vi "PROGRAMA.vi"() -> ()   [LabVIEW 2011]
doc: "Read one the value of one analog channel from a LINX device."
uses:
  <vilib>/Platform/TimedLoop/XDataNode/timing_clust.ctl
  <vilib>/Platform/TimedLoop/XDataNode/nitl_modes.ctl
  <vilib>/Platform/TimedLoop/XDataNode/wakeup.ctl
  <vilib>/MakerHub/LINX/Public/Peripherals/Analog/Analog Read 1 Chan.vi
  <vilib>/MakerHub/LINX/Public/Peripherals/PWM/PWM Set Duty Cycle 1 Chan.vi
  <vilib>/MakerHub/LINX/Public/Peripherals/Digital/Digital Write 1 Chan.vi
  <vilib>/MakerHub/LINX/Public/Peripherals/Analog/Analog Read N Chans.vi
  <vilib>/MakerHub/LINX/Public/Peripherals/Digital/Digital Write N Chans.vi
  <vilib>/MakerHub/LINX/Private/Local IO/LinxAnalogRead.vi
  <vilib>/MakerHub/LINX/Public/Utilities/Check Channel.vi
  <vilib>/MakerHub/LINX/Private/Local IO/LinxDigitalWrite.vi
  <vilib>/MakerHub/LINX/Public/Utilities/Open Serial.vi
  <vilib>/addons/Fuzzy Logic/FL Fuzzy Controller (SISO).vi
  <vilib>/addons/Fuzzy Logic/FL Fuzzy Controller (SIMO).vi
  <vilib>/addons/control/pid/pid.llb/PID (DBL).vi
  <vilib>/Utility/file.llb/Write To Spreadsheet File (string).vi
  <vilib>/MakerHub/LINX/Private/Utilties/Generate Error.vi
  <vilib>/Utility/file.llb/Read From Spreadsheet File (DBL).vi
  <vilib>/MakerHub/LINX/Public/Peripherals/PWM/PWM Set Duty Cycle N Chans.vi
  <vilib>/Platform/TimedLoop/XDataNode/XDataNode.xnode
  <vilib>/express/express arith-compare/Formula/XNode/ExpressFormulaBlockNode.xnode
  <vilib>/MakerHub/LINX/LMH-LINX.lvlib
  <vilib>/addons/Fuzzy Logic/NI_Fuzzy_Logic_API.lvlib
  <vilib>/addons/control/pid/NI_PID_pid.lvlib
  <vilib>/Platform/TimedLoop/XDataNode/XDNodeRunTimeDep.lvlib
panel:
  out "BOMBA":dbl format="%.0p%%"
  out "AC. VÁLVULAS":dbl
  out "MSE":dbl
  in  "Tempo Derivativo (Td)":dbl=0.00014 min=0.0 max=25.0 step=1e-05 format="%.6g"
  in  "Tempo de Integração (Ti)":dbl=0.002 min=0.0 max=25.0 step=1e-05 format="%.6g"
  in  "ZN/Manual":bool
  in  "Ganho Proporcional (Kp)":dbl=15.0 min=0.0 max=15.0 format="%.6g"
  out "Ganhos - ZN/Manual":T1={"Ganho Proporcional (Kp)"=1.9838195929127882, "Tempo de Integração (Ti)"=0.01995856284686879, "Tempo Derivativo (Td)"=0.0} {"Tempo Derivativo (Td)" format="%#.6g"; "Tempo de Integração (Ti)" format="%#.6g"; "Ganho Proporcional (Kp)" format="%#.6g"}
  in  "Ganhos do PID":bool
  out "Ganhos - Fuzzy":T1={"Ganho Proporcional (Kp)"=1.9838195929127882, "Tempo de Integração (Ti)"=0.01995856284686879, "Tempo Derivativo (Td)"=0.0} {"Tempo Derivativo (Td)" format="%#.6g"; "Tempo de Integração (Ti)" format="%#.6g"; "Ganho Proporcional (Kp)" format="%#.6g"}
  out "GRAFICO":cluster{"Set-Point":dbl, dbl, dbl, dbl, dbl}(graph)
  in  "AUTO":bool
  out "Erro":dbl
  in  "Set-Point":dbl=30.0 min=15.0 max=150.0 step=1.0
  out "Porta-Saída-Válvula-3":dbl
  out "Porta-Saída-Válvula-2":dbl
  out "Porta-Saída-Válvula-1":dbl
  out "Porta-Leitura-5VCC":dbl
  out "Porta-Saída-Bomba":dbl
  out "Porta-Sensor-Pressão":dbl
  out "Pressão (mmHg)":dbl
  in  "V1":bool
  in  "V3":bool
  in  "V2":bool
  in  "Controle - bomba (%)":dbl(slide) scale=0.0..100.0
  out "Loop Rate (Hz)":u32
  in  "Stop Button":bool
  in  "Serial Port":refnum<visa-resource-name>
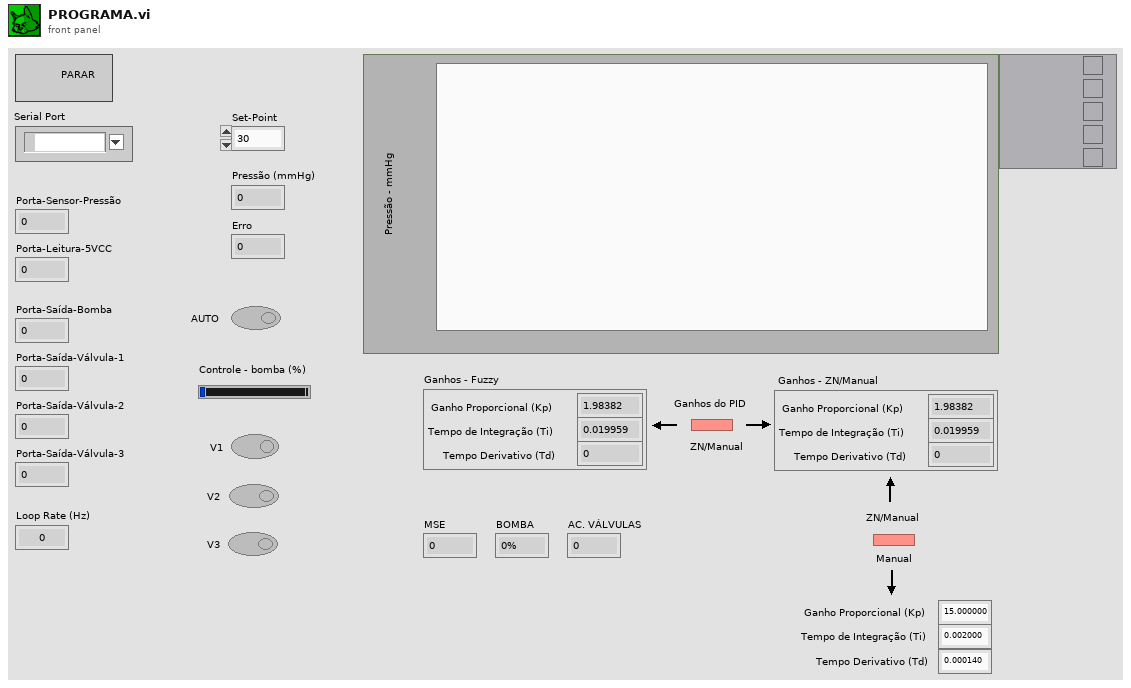
[diagram p1: front panel]
types:
  T1 = cluster{"Ganho Proporcional (Kp)":dbl, "Tempo de Integração (Ti)":dbl, "Tempo Derivativo (Td)":dbl}
  T2 = typedef "LMH-LINX.lvlib/LINX Ref.ctl" = cluster{"IO":T3, "Interface":T4, "LINX Device Config":T5}
  T3 = typedef "LMH-LINX.lvlib/Platform.ctl" = enum16{"Remote", "Local"}
  T4 = typedef "LMH-LINX.lvlib/Interface.ctl" = enum16{"Serial", "TCP"}
  T5 = typedef "LMH-LINX.lvlib/Device.lvlib/LINX Device Config.ctl" = cluster{"Interface":T4, "COM Port":refnum<visa-resource-name>, "TCP Configuration":T6, "Device Family":u8, "Device ID":u8, "Device Name":string, "TCP Ref":refnum<k5>, "Channels":T7}
  T6 = typedef "LMH-LINX.lvlib/Device.lvlib/TCP Config.ctl" = cluster{"IP Address":string, "Port":u16}
  T7 = typedef "LMH-LINX.lvlib/Channels.ctl" = cluster{"DI":u8[], "DO":u8[], "AI":u8[], "AO":u8[], "PWM":u8[], "QE":u8[], "UART":u8[], "I2C 2":u8[], "SPI":u8[], "CAN":u8[], "Servo":u8[], "AI Ref (V)":dbl, "AI Resolution (Bits)":u8, "AO Ref (V)":dbl, "AO Resolution (Bits)":u8}
  T8 = typedef "NI_Fuzzy_Logic_API.lvlib/FL System.ctl" = cluster{"input variables":T9[], "output variables":T9[], "rules":T12[], "defuzzification method":T18, "description":string, "user MF interpolating polynomials":T19[]}
  T9 = typedef "NI_Fuzzy_Logic_API.lvlib/FL Variable.ctl" = cluster{"name":string, "range":dbl[], "MFs":T10[]}
  T10 = typedef "NI_Fuzzy_Logic_API.lvlib/FL Membership Function.ctl" = cluster{"name":string, "shape":T11, "points":dbl[], "color":u32, "user-defined shape index":i32}
  T11 = typedef "NI_Fuzzy_Logic_API.lvlib/FL Membership Function Shape.ctl" = u16
  T12 = typedef "NI_Fuzzy_Logic_API.lvlib/FL Rule.ctl" = cluster{"antecedents":T13[], "antecedent connective":T15, "consequents":T16[], "consequent implication":T17, "degree of support":dbl}
  T13 = typedef "NI_Fuzzy_Logic_API.lvlib/FL Antecedent.ctl" = cluster{"Var Index":i32, "MF Index":i32, "Cond":T14}
  T14 = typedef "FL Modifier.ctl" = u16
  T15 = typedef "NI_Fuzzy_Logic_API.lvlib/FL Antecedent Connective.ctl" = u16
  T16 = typedef "NI_Fuzzy_Logic_API.lvlib/FL Consequent.ctl" = cluster{"Var Index":i32, "MF Index":i32, "Cond":T14}
  T17 = typedef "NI_Fuzzy_Logic_API.lvlib/FL Consequent Implication.ctl" = u16
  T18 = typedef "NI_Fuzzy_Logic_API.lvlib/FL Defuzzification.ctl" = u16
  T19 = typedef "NI_Fuzzy_Logic_API.lvlib/FL Interpolating polynomials.ctl" = cluster{"X":dbl[], "Y":dbl[], "Y(x) coeff":dbl[][], "X(y) coeff":dbl[][], "Area(y) coeff":dbl[][], "coa_x(y) coeff":dbl[][]}
  T20 = typedef "XDNodeRunTimeDep.lvlib/timing_clust.ctl" = cluster{"Expected End [f-1]":u64, "Actual End [f-1]":u64, "Finished Late? [f-1]":bool, "Expected End [i-1]":u64, "Actual End [i-1]":u64, "Finished Late? [i-1]":bool, "Expected Start [i]":u64, "Actual Start [i]":u64, "Expected Start [f]":u64, "Actual Start [f]":u64, "Source Name":string, "Structure Name":string, "Period":i64, "Deadline":i64, "Offset":i64, "Start":i64, "Priority":i32, "Timeout":i32, "Mode":T21, "Wakeup Reason":T22, "Error":errorcluster, "Source Type":string, "Secondary Source Type":string, "Global End Time":u64, "Global Start Time":u64, "Frame Duration":u64, "Iteration Duration":u64, "Assigned CPU":i32, "I/O Scan Engine Mode":u32}
  T21 = typedef "XDNodeRunTimeDep.lvlib/nitl_modes.ctl" = enum32{"No Change", "Process missed periods, maintain original phase", "Discard missed periods, maintain original phase", "Process missed periods, ignore original phase", "Discard missed periods, ignore original phase"}
  T22 = typedef "XDNodeRunTimeDep.lvlib/wakeup.ctl" = enum32{"Normal", "Aborted", "Asynchronous wakeup", "Timing source error", "Timed loop error", "Timeout"}
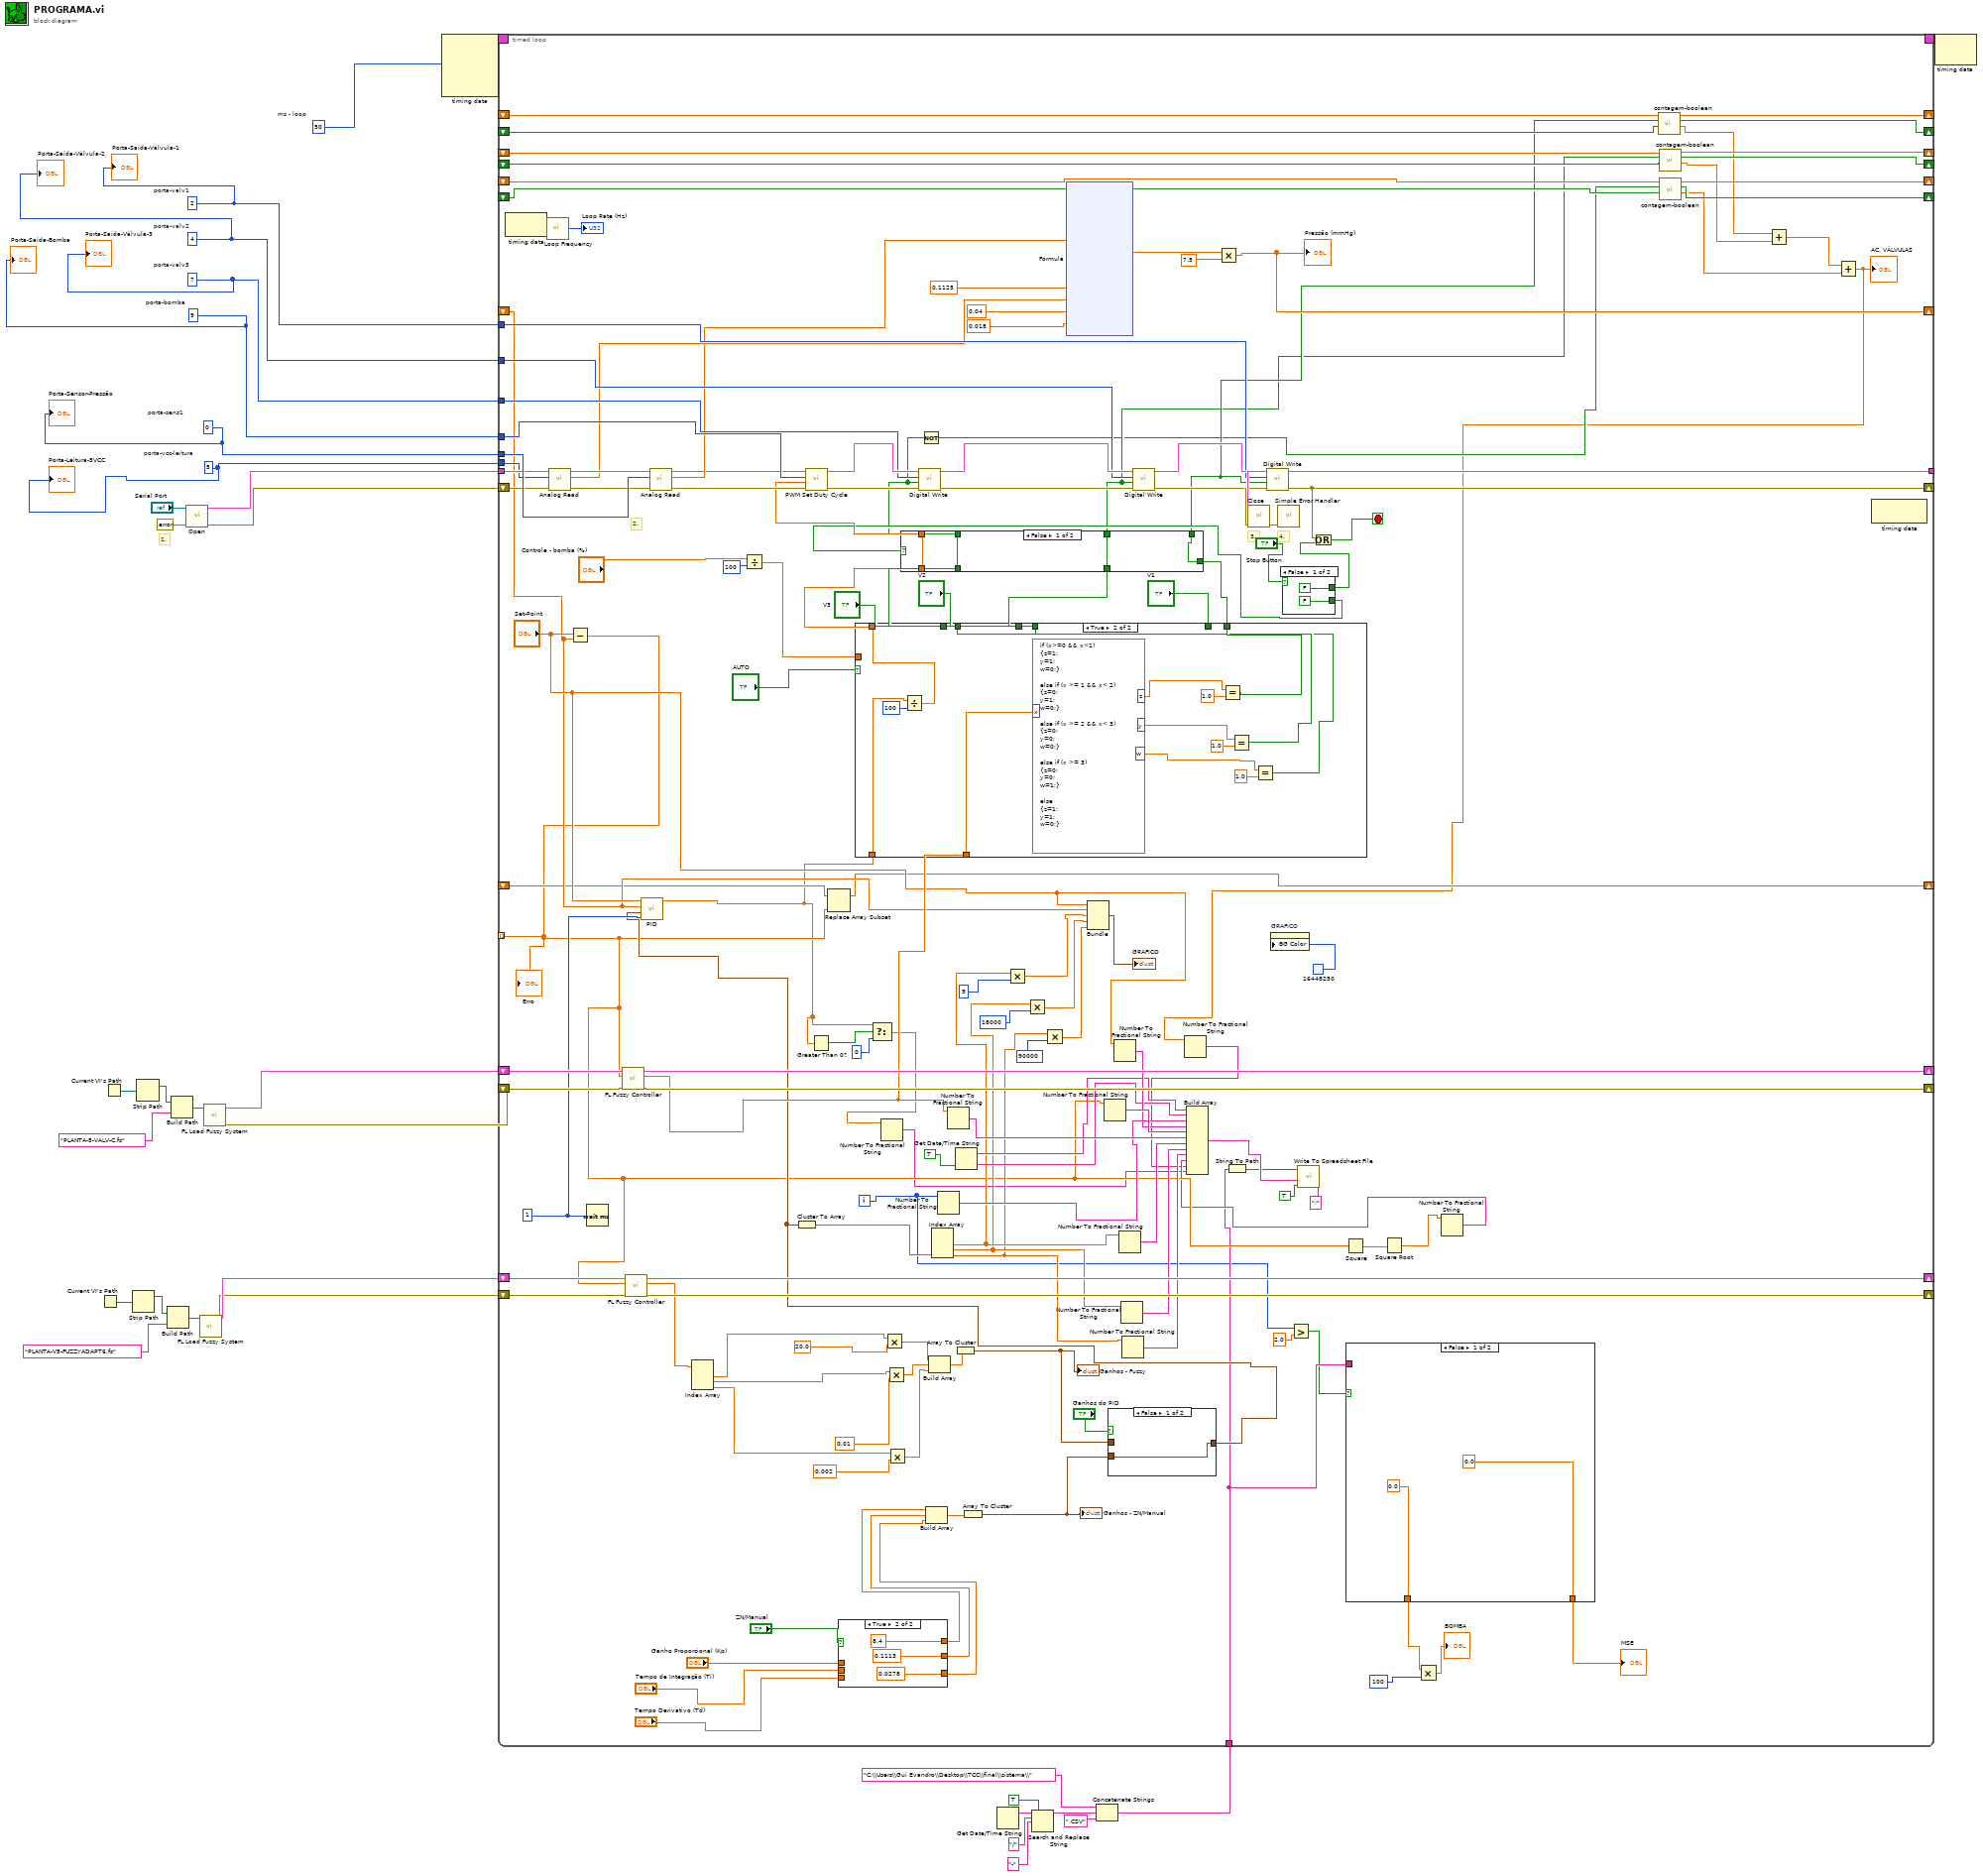
[diagram p0: block diagram]
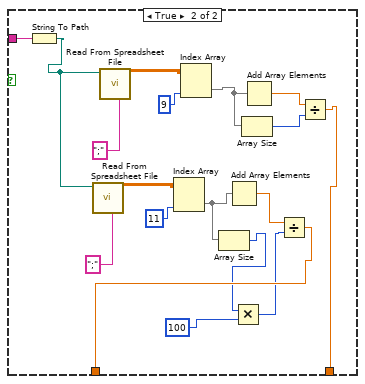
[diagram p2: hidden frame]
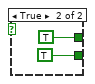
[diagram p3: hidden frame]
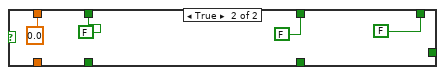
[diagram p4: hidden frame]
diagram:
  w9 = 50  # ms - loop
  w28 = 5  # porta-vcc-leitura
  w29 = 0  # porta-sens1
  w27 = 2  # porta-valv1
  w26 = 4  # porta-valv2
  w25 = 7  # porta-valv3
  w24 = 9  # porta-bomba
  # "4."
  # "3."
  # "1."
  n1 = Current VI's Path() -> (path=w17:path)
  n2 = Current VI's Path() -> (path=w20:path)
  n3 = Strip Path(path=w17) -> (stripped path=w16:path)  [unwired: 1 out]
  n4 = Strip Path(path=w20) -> (stripped path=w21:path)  [unwired: 1 out]
  n5 = Build Path(base path=w16, name or relative path="PLANTA-V5-FUZZYADAPT6.fs") -> (appended path=w14:path)
  n6 = Build Path(base path=w21, name or relative path="PLANTA-5-VALV-C.fs") -> (appended path=w23:path)
  n7 = call-poly <vilib>:"Open.vi"("Error In"=errorcluster {"status"=FALSE, "code"=0, "source"=""}, "Serial Port"="Serial Port") -> ("Error Out"=w30:errorcluster, "LINX Resource"=w31:T2)  [unwired: 7 in, 1 out]
  n8 = call <vilib>:"FL Load Fuzzy System.vi"("file path"=w14) -> ("error out"=w12:errorcluster, "fuzzy system out"=w13:T8)  [unwired: 1 in, 8 out]
  n9 = call <vilib>:"FL Load Fuzzy System.vi"("file path"=w23) -> ("error out"=w18:errorcluster, "fuzzy system out"=w19:T8)  [unwired: 1 in, 8 out]
  n10 = node-c288(w9) -> (w11:T20)  [unwired: 3 in]
  n11 = Get Date/Time String() -> (date string=w6:string)  [unwired: 3 in, 1 out]
  n12 = Search and Replace String(replace all?=TRUE, input string=w6, search string="/", replace string="-") -> (result string=w3:string)  [unwired: 4 in, 3 out]
  n13 = Concatenate Strings("C:\\Users\\Gui Evandro\\Desktop\\TCC\\final\\sistema\\", w3, ".CSV") -> (w1:string)
  n14 = timed-loop {
    tunnel: w31 -> [w163]
    tunnel: [w170] -> w36
    shift-right: [w173] -> w35
    shift-left: w30 -> [w164]
    tunnel: w29 -> [w181]
    tunnel: w24 -> [w180]
    tunnel: w25 -> [w177]
    tunnel: w26 -> [w174]
    tunnel: w27 -> [w169]
    tunnel: w28 -> [w162]
    shift-right: [w149] -> _
    shift-left: w19 -> [w150]
    shift-right: [w148] -> _
    shift-left: w18 -> [w147]
    shift-right: [w144] -> _
    shift-left: _ -> [w79]
    tunnel: w1 -> [w71]
    shift-right: [w136] -> _
    shift-left: w13 -> [w138]
    shift-right: [w135] -> _
    shift-left: w12 -> [w137]
    timing: w11 -> [_]
    timing-out: [_] -> w10
    tunnel: [w75] -> _ mode=indexing
    shift-right: [w76] -> _
    shift-left: _ -> [w77]
    shift-right: [w65] -> _
    shift-left: _ -> [w62]
    shift-right: [w63] -> _
    shift-left: _ -> [w60]
    shift-right: [w64] -> _
    shift-left: _ -> [w61]
    shift-right: [w55] -> _
    shift-left: _ -> [w54]
    shift-right: [w56] -> _
    shift-left: _ -> [w58]
    shift-right: [w57] -> _
    shift-left: _ -> [w59]
    i -> [w70]
    stop <- w183 stop-if-true
    w139 = u32 1 ("milliseconds to wait")
    # "2."
    n15 = node-c288() -> ()  [unwired: 1 in, 1 out]
    n16 = call <vilib>:"Loop Frequency.vi"() -> ("Loop Rate (Hz)"=→"Loop Rate (Hz)":u32)
    n17 = call-poly <vilib>:"Analog Read.vi"("Error In"=w164, "Analog Channel"=w162, "LINX Resource"=w163) -> ("Error Out"=w165:errorcluster, "Voltage"=w158:dbl, "LINX Resource"=w166:T2)  [unwired: 5 in, 1 out]
    n18 = Subtract(x="Set-Point", y=w79) -> (x-y=w75:dbl)
    "Erro" <- w75
    n19 = Wait (ms)(milliseconds to wait=w139) -> ()  [unwired: 1 out]
    n20 = call-poly <vilib>:"FL Fuzzy Controller.vi"("error in (no error)"=w147, "input value"=w75, "fuzzy system in"=w150) -> ("error out"=w148:errorcluster, "output value"=w104:dbl, "fuzzy system out"=w149:T8)  [unwired: 6 out]
    n21 = call-poly <vilib>:"FL Fuzzy Controller.vi"("error in (no error)"=w137, "input value"=w75, "fuzzy system in"=w138) -> ("error out"=w135:errorcluster, "output values"=w133:dbl[], "fuzzy system out"=w136:T8)  [unwired: 6 out]
    n22 = call-poly <vilib>:"Analog Read.vi"("Error In"=w165, "Analog Channel"=w181, "LINX Resource"=w166) -> ("Error Out"=w153:errorcluster, "Voltage"=w155:dbl, "LINX Resource"=w154:T2)  [unwired: 5 in, 1 out]
    n23 = Index Array(array=w133) -> (element #1=w132:dbl, element #2=w131:dbl, element #3=w130:dbl)  [unwired: 3 in]
    n24 = Divide(x="Controle - bomba (%)", y=100) -> (x/y=w151:dbl)
    n25 = Replace Array Subset(array=w77, new element=w75) -> (w76:dbl[])  [unwired: 1 in]
    n26 = case shown="True" "ZN/Manual" {
      tunnel: [w220 8.4 ("E")] -> w119
      tunnel: [w219 0.1113 ("E")] -> w118
      tunnel: [w218 0.0278 ("E")] -> w117
      tunnel: "Ganho Proporcional (Kp)" -> [w220 _]
      tunnel: "Tempo de Integração (Ti)" -> [w219 _]
      tunnel: "Tempo Derivativo (Td)" -> [w218 _]
      frame False {
      }
      frame True {
      }
    }
    n27 = Multiply(x=w132, y=20.0 ("E")) -> (x*y=w126:dbl)
    n28 = Multiply(x=w131, y=0.01 ("E")) -> (x*y=w125:dbl)
    n29 = Multiply(x=w130, y=0.002 ("E")) -> (x*y=w124:dbl)
    n30 = Build Array(w119, w118, w117) -> (w121:dbl[])
    n31 = Build Array(w126, w125, w124) -> (w134:dbl[])
    n32 = Number To Fractional String(number=w70) -> (F-format string=w101:string)  [unwired: 3 in]
    n33 = Number To Fractional String(number=w104) -> (F-format string=w103:string)  [unwired: 3 in]
    n34 = Array To Cluster(array=w134) -> (cluster=w122:cluster{"[0]":dbl, "[1]":dbl, "[2]":dbl})
    "Ganhos - Fuzzy" <- w122
    n35 = Get Date/Time String(want seconds? (F)=TRUE) -> (date string=w99:string, time string=w98:string)  [unwired: 2 in]
    n36 = Array To Cluster(array=w121) -> (cluster=w115:cluster{"[0]":dbl, "[1]":dbl, "[2]":dbl})
    "Ganhos - ZN/Manual" <- w115
    n37 = xnode "Formula"("V"=w155, "E"=0.1125, "A"=w158, "C"=0.04, "B"=0.018) -> ("Result"=w157:dbl)  [unwired: 1 in, 1 out]
    n38 = Number To Fractional String(number=w75) -> (F-format string=w102:string)  [unwired: 3 in]
    n39 = case shown="False" "Ganhos do PID" {
      tunnel: w122 -> [_ w225]
      tunnel: [w224 w225] -> w92
      tunnel: w115 -> [w224 _]
      frame False {
      }
      frame True {
      }
    }
    n40 = call-poly <vilib>:"PID.vi"("dt (s)"=w139, "PID gains"=w92, "process variable"=w79, "setpoint"="Set-Point") -> ("output"=w44:dbl)  [unwired: 6 in, 1 out]
    n41 = Cluster To Array(cluster=w92) -> (array=w91:dbl[])
    n42 = Greater Than 0?(x=w44) -> (x > 0?=w45:bool)
    n43 = case shown="True" "AUTO" {
      tunnel: [w229 w241] -> w109
      tunnel: w151 -> [w229 _]
      tunnel: w104 -> [_ w239]
      tunnel: [w228 w232] -> w110
      tunnel: "V1" -> [w228 _]
      tunnel: [w227 w231] -> w111
      tunnel: "V2" -> [w227 _]
      tunnel: w44 -> [_ w240]
      tunnel: "V3" -> [w226 _]
      tunnel: [w226 w230] -> w112
      frame False {
      }
      frame True {
        n44 = Divide(x=w240, y=100) -> (x/y=w241:dbl)
        n45 = formula code="if (x>=0 && x<1)\n{z=1;\ny=1;\nw=0;}\n\nelse if (x >= 1 && x< 2)\n{z=0;\ny=1;\nw=0;}\n\nelse if (x >= 2 && x< 3)\n{z=0;\ny=0;\nw=0;}\n\nelse if (x >= 3)\n{z=0;\ny=0;\nw=1;}\n\nelse\n{z=1;\ny=1;\nw=0;}"("x"=w239) -> ("z"=w235:dbl, "y"=w234:dbl, "w"=w233:dbl)
        n46 = Equal?(x=w235, y=1.0) -> (x = y?=w232:bool)
        n47 = Equal?(x=w234, y=1.0) -> (x = y?=w231:bool)
        n48 = Equal?(x=w233, y=1.0) -> (x = y?=w230:bool)
      }
    }
    n49 = Select(t=w44, s=w45, f=0) -> (s? t:f=w37:dbl)
    n50 = Number To Fractional String(number=w37) -> (F-format string=w42:string)  [unwired: 3 in]
    n51 = Index Array(array=w91) -> (element #1=w87:dbl, element #2=w86:dbl, element #3=w85:dbl)  [unwired: 3 in]
    n52 = Multiply(x=w87, y=9) -> (x*y=w83:dbl)
    n53 = Multiply(x=w86, y=18000) -> (x*y=w82:dbl)
    n54 = Multiply(x=w85, y=90000) -> (x*y=w81:dbl)
    n55 = Bundle("Set-Point"="Set-Point", w79, w83, w82, w81) -> (→"GRAFICO":cluster{"Set-Point":dbl, dbl, dbl, dbl, dbl})  [unwired: 1 in]
    n56 = Number To Fractional String(number="Set-Point") -> (F-format string=w100:string)  [unwired: 3 in]
    n57 = Number To Fractional String(number=w87) -> (F-format string=w96:string)  [unwired: 3 in]
    n58 = Number To Fractional String(number=w86) -> (F-format string=w95:string)  [unwired: 3 in]
    n59 = Number To Fractional String(number=w85) -> (F-format string=w94:string)  [unwired: 3 in]
    n60 = Multiply(x=w157, y=7.5) -> (x*y=w144:dbl)
    "Pressão (mmHg)" <- w144
    n61 = String To Path(string=w71) -> (path=w78:path)
    n62 = property on="GRAFICO" class="WFChart (strict)"("BG Color"=u32 16448250) -> ()  [unwired: 2 in, 2 out]
    n63 = case shown="False" "Stop Button" {
      tunnel: [FALSE TRUE] -> w106
      tunnel: [FALSE TRUE] -> w105
      frame False {
      }
      frame True {
      }
    }
    n64 = case shown="False" w105 {
      tunnel: w112 -> [w213 _]
      tunnel: [w213 FALSE] -> w66
      tunnel: w111 -> [w212 _]
      tunnel: [w212 FALSE] -> w52
      tunnel: w110 -> [w211 _]
      tunnel: [w211 FALSE] -> w53
      tunnel: w109 -> [w210 _]
      tunnel: [w210 0.0] -> w108
      frame False {
      }
      frame True {
      }
    }
    n65 = call-poly <vilib>:"PWM Set Duty Cycle.vi"("Error In"=w153, "Duty Cycle (0-1)"=w108, "PWM Channel"=w180, "LINX Resource"=w154) -> ("Error Out"=w178:errorcluster, "LINX Resource"=w179:T2)  [unwired: 6 in]
    n66 = call-poly <vilib>:"Digital Write.vi"("Error In"=w178, "Output Value"=w66, "DO Channel"=w177, "LINX Resource"=w179) -> ("Error Out"=w175:errorcluster, "LINX Resource"=w176:T2)  [unwired: 6 in]
    n67 = Not(x=w66) -> (.not. x?=w51:bool)
    n68 = call-poly <vilib>:"Digital Write.vi"("Error In"=w175, "Output Value"=w52, "DO Channel"=w174, "LINX Resource"=w176) -> ("Error Out"=w172:errorcluster, "LINX Resource"=w171:T2)  [unwired: 6 in]
    n69 = call-poly <vilib>:"Digital Write.vi"("Error In"=w172, "Output Value"=w53, "DO Channel"=w169, "LINX Resource"=w171) -> ("Error Out"=w173:errorcluster, "LINX Resource"=w170:T2)  [unwired: 6 in]
    n70 = Greater?(x=w70, y=2.0 ("E")) -> (0:w68:bool)
    n71 = Or(x=w173, y=w106) -> (x .or. y?=w183:bool)
    n72 = Square(x=w75) -> (x^2=w74:dbl)
    n73 = case shown="False" w68 {
      tunnel: [0.0 ("E") w197] -> w38
      tunnel: w71 -> [_ w196]
      tunnel: [0.0 ("E") w189] -> w40
      frame False {
      }
      frame True {
        n74 = String To Path(string=w196) -> (path=w192:path)
        n75 = call-poly <vilib>:"Read From Spreadsheet File.vi"("delimiter (\\t)"=";", "file path (dialog if empty)"=w192) -> ("all rows"=w194:dbl[][])  [unwired: 5 in, 4 out]
        n76 = call-poly <vilib>:"Read From Spreadsheet File.vi"("delimiter (\\t)"=";", "file path (dialog if empty)"=w192) -> ("all rows"=w200:dbl[][])  [unwired: 5 in, 4 out]
        n77 = Index Array(array=w194, index (col)=11 ("disabled index (col)")) -> (element=w191:dbl[])  [unwired: 1 in]
        n78 = Index Array(array=w200, index (col)=9 ("disabled index (col)")) -> (element=w198:dbl[])  [unwired: 1 in]
        n79 = Array Size(array=w191) -> (size(s)=w188:i32)
        n80 = Add Array Elements(numeric array=w191) -> (sum=w190:dbl)
        n81 = Multiply(x=w188, y=100 ("disabled index (col)")) -> (x*y=w186:i32)
        n82 = Array Size(array=w198) -> (size(s)=w202:i32)
        n83 = Add Array Elements(numeric array=w198) -> (sum=w203:dbl)
        n84 = Divide(x=w190, y=w186) -> (x/y=w189:dbl)
        n85 = Divide(x=w203, y=w202) -> (x/y=w197:dbl)
      }
    }
    "MSE" <- w38
    n86 = Square Root(x=w74) -> (sqrt(x)=w73:dbl)
    n87 = Multiply(x=w40, y=100 ("disabled index (col)")) -> (x*y=→"BOMBA":dbl)
    n88 = Number To Fractional String(number=w73) -> (F-format string=w72:string)  [unwired: 3 in]
    n89 = call "contagem-boolean.vi"("Boolean 2"=w54, "Boolean"=w53, "Numeric in"=w60) -> ("contage 2"=w49:dbl, "Boolean 3"=w55:bool, "Numeric out"=w63:dbl)  [unwired: 6 in]
    n90 = call "contagem-boolean.vi"("Boolean 2"=w58, "Boolean"=w52, "Numeric in"=w61) -> ("contage 2"=w48:dbl, "Boolean 3"=w56:bool, "Numeric out"=w64:dbl)  [unwired: 6 in]
    n91 = call "contagem-boolean.vi"("Boolean 2"=w59, "Boolean"=w51, "Numeric in"=w62) -> ("contage 2"=w47:dbl, "Boolean 3"=w57:bool, "Numeric out"=w65:dbl)  [unwired: 6 in]
    n92 = Add(x=w49, y=w48) -> (x+y=w50:dbl)
    n93 = Add(x=w50, y=w47) -> (x+y=w46:dbl)
    "AC. VÁLVULAS" <- w46
    n94 = Number To Fractional String(number=w46) -> (F-format string=w67:string)  [unwired: 3 in]
    n95 = Build Array(w99, w98, w101, w100, w102, w103, w96, w95, w94, w72, w67, w42) -> (w141:string[])
    n96 = call-poly <vilib>:"Write To Spreadsheet File.vi"("delimiter (\\t)"=";", "append to file? (new file:F)"=TRUE, "1D data"=w141, "file path (dialog if empty)"=w78) -> ()  [unwired: 4 in, 1 out]
    n97 = node-c288() -> ()  [unwired: 1 in, 1 out]
  }
  n98 = call <vilib>:"Close.vi"("Error In"=w35, "LINX Resource"=w36) -> ("Error Out"=w33:errorcluster)  [unwired: 9 in]
  n99 = call <vilib>:"Simple Error Handler.vi"("error in (no error)"=w33) -> ()  [unwired: 4 in, 5 out]
  n100 = node-c288(w10) -> ()  [unwired: 1 out]
  "Porta-Sensor-Pressão" <- w29
  "Porta-Saída-Bomba" <- w24
  "Porta-Leitura-5VCC" <- w28
  "Porta-Saída-Válvula-1" <- w27
  "Porta-Saída-Válvula-2" <- w26
  "Porta-Saída-Válvula-3" <- w25
